vi "Poly_Two_Button.vi"(8 "error in":errorcluster, 9 "Button 2 Text":string, 10 "Button 1 Text":string, 11 "Message":string) -> (0 "error out":errorcluster, 3 "OK":bool)   [LabVIEW 2024, in "Launcher_DTU.lvlib"]
uses:
  Launcher_DTU.lvlib
panel:
  out "Message":string
  in  "Button 2":bool
  in  "Button 1":bool
  # "Attention !"
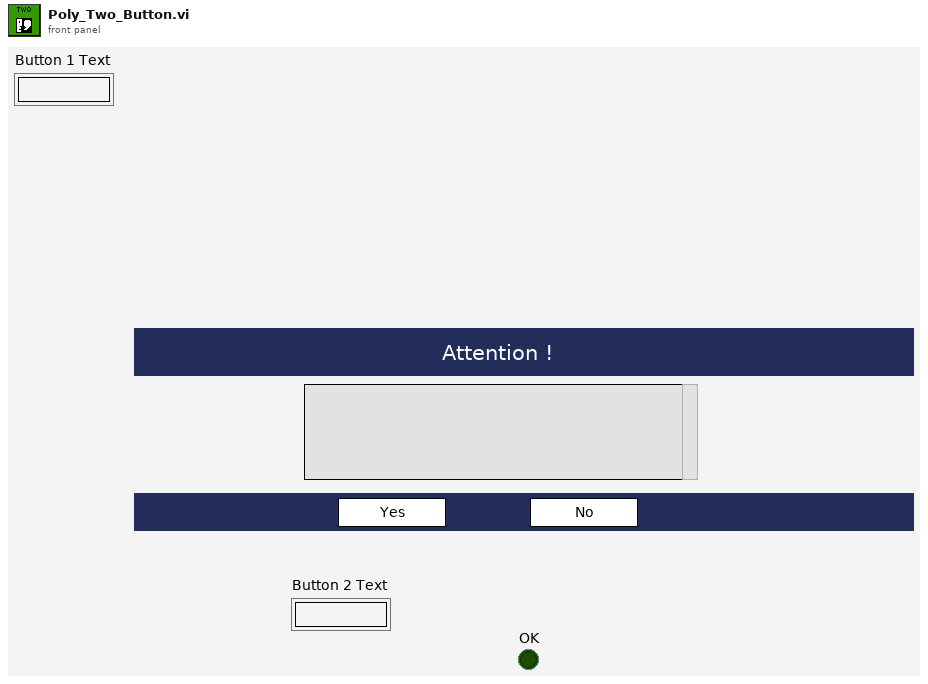
[diagram p1: front panel]
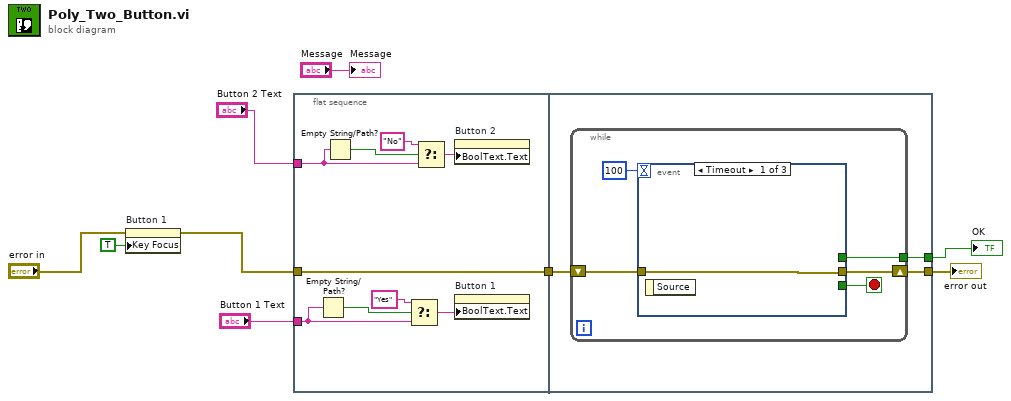
[diagram p0: block diagram]
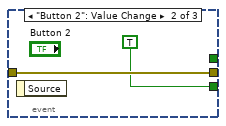
[diagram p2: hidden frame]
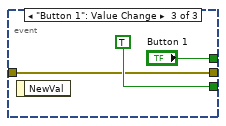
[diagram p3: hidden frame]
diagram:
  n1 = property on="Button 1" class="Bool"(error in="error in", "Key Focus"=TRUE) -> (error out=w1:errorcluster)  [unwired: 1 in, 1 out]
  n2 = flat-sequence {
    tunnel: [w18] -> w8
    tunnel: w1 -> [w18]
    tunnel: "Button 1 Text" -> [w16]
    tunnel: "Button 2 Text" -> [w10]
    tunnel: [w21] -> w9
    tunnel: w8 -> [w20]
    tunnel: [w19] -> w6
    frame #0 {
      n3 = Empty String/Path?(string/path=w16) -> (empty?=w17:bool)
      n4 = Empty String/Path?(string/path=w10) -> (empty?=w12:bool)
      n5 = Select(t="Yes", s=w17, f=w16) -> (s? t:f=w15:string)
      n6 = Select(t="No", s=w12, f=w10) -> (s? t:f=w11:string)
      n7 = property on="Button 2" class="Bool"("BoolText.Text"=w11) -> ()  [unwired: 2 in, 2 out]
      n8 = property on="Button 1" class="Bool"("BoolText.Text"=w15) -> ()  [unwired: 2 in, 2 out]
    }
    frame #1 {
      n9 = while {
        shift-right: [w24] -> w21
        shift-left: w20 -> [w25]
        tunnel: [w23] -> w19
        stop <- w22 stop-if-true
        n10 = event shown="[0] Timeout" {
          selector: _ -> [_ _ _]
          dyn-events: _ -> [_ _ _]
          timeout: 100 -> [_ _ _]
          tunnel: [_ TRUE TRUE] -> w22
          tunnel: w25 -> [w27 w29 w31]
          tunnel: [w27 w29 w31] -> w24
          tunnel: [_ _ "Button 1"] -> w23
          event Timeout {
            n11 = event-data() -> ()  [unwired: 1 in, 1 out]
          }
          event "Button 2": Value Change {
            n12 = event-data() -> ()  [unwired: 1 in, 1 out]
          }
          event "Button 1": Value Change {
            n13 = event-data() -> ()  [unwired: 1 in, 1 out]
          }
        }
      }
    }
  }
  "error out" <- w9
  "OK" <- w6
  "Message" <- "Message"
